vi "Instantiate Py Doc.vi"(5 "Py File Path":path, 11 "error in (no error)":errorcluster) -> (4 "Document out":refnum<class "Document.lvclass">, 15 "error out":errorcluster)   [LabVIEW 2016, in "Py Doc.lvclass"]
uses:
  Py Doc.lvclass
  Document.lvclass
  C:/Users/namratha.balakrishna/Desktop/source code/MDI/D/MDI Project/source code/Document/Document.lvclass
  Document.lvclass/Document.ctl
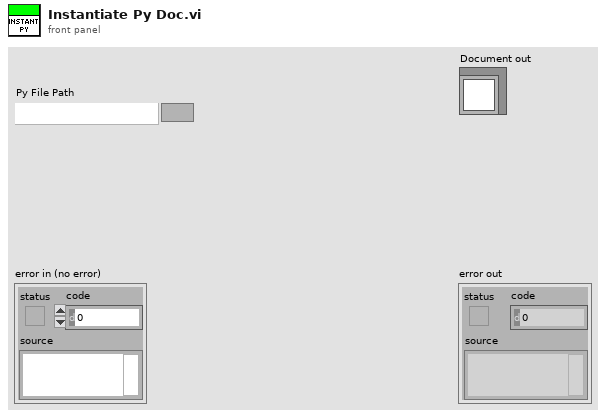
[diagram p1: front panel]
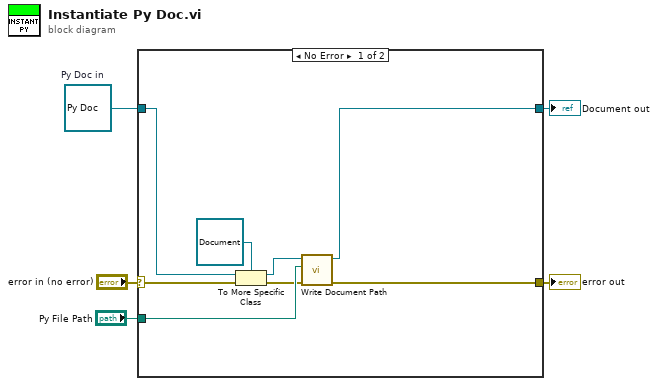
[diagram p0: block diagram]
diagram:
  w3 = refnum<class "Py Doc.lvclass"> refnum  # Py Doc in
  n1 = case shown="No Error" "error in (no error)" {
    selector: "error in (no error)" -> [w12 w15]
    tunnel: [w10 w15] -> w4
    tunnel: [w9 w14] -> w1
    tunnel: w3 -> [w13 w14]
    tunnel: "Py File Path" -> [w11 _]
    frame No Error {
      n2 = To More Specific Class(target class=refnum<class "Document.lvclass"> refnum ("Document.lvclass"), reference=w13, error in=w12) -> (specific class reference=w7:refnum<class "Document.lvclass">, error out=w6:errorcluster)
      n3 = call "Write Document Path.vi"("error in (no error)"=w6, "Document Path"=w11, "Document in"=w7) -> ("error out"=w10:errorcluster, "Document out"=w9:refnum<class "Document.lvclass">)  [unwired: 7 in]
    }
    frame Error {
    }
  }
  "error out" <- w4
  "Document out" <- w1
